vi "AlliGator Get-Set TIFF Series Options.vi"(6 "Set/Get (F)":bool, 8 "error in (no error)":errorcluster, 11 "output cluster in":T1) -> (0 "error out":errorcluster, 3 "output cluster out":T1)   [LabVIEW 2021, in "AlliGator Files.lvlib"]
doc: "Storage of options for dataset export to TIFF series."
uses:
  AlliGator Files.lvlib
  AlliGator TIFF Series Options.ctl
panel:
  # "see the AlliGator License on the block diagram (Ctrl+E or Window:Show Block Diagram)"
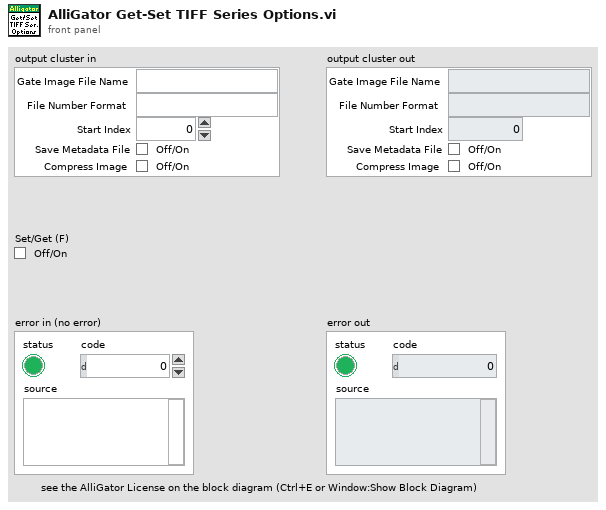
[diagram p1: front panel]
types:
  T1 = typedef "AlliGator Files.lvlib/AlliGator TIFF Series Options.ctl" = cluster{"Gate Image File Name":string, "File Number Format":string, "Start Index":u32, "Save Metadata File":bool, "Compress Image":bool}
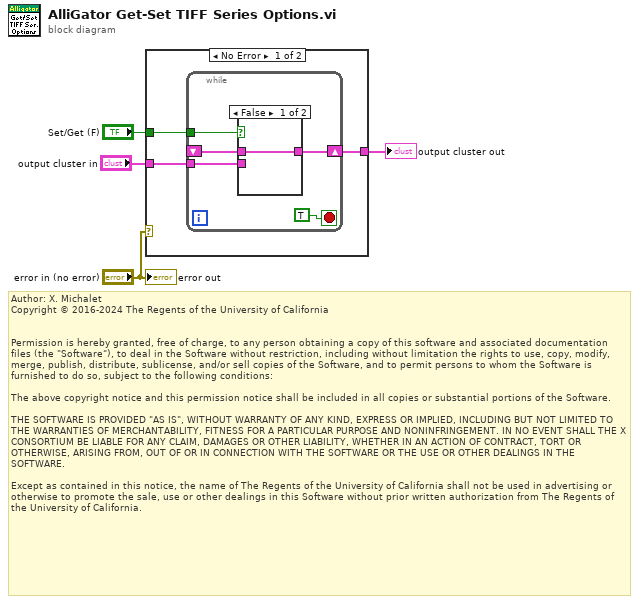
[diagram p0: block diagram]
diagram:
  # "Author: X. Michalet\nCopyright © 2016-2024 The Regents of the University of California\n \n\nPermission is hereby granted, free of charge, to any person obtaining a copy of this software and associated documentation files (the \"Software\"), to deal in the Software without restriction, including without limitation the rights to use, copy, modify, merge, publish, distribute, sublicense, and/or sell copies of the Software, and to permit persons to whom the Software is furnished to do so, subject to the following conditions:\n\nThe above copyright notice and this permission notice shall be included in all copies or substantial portions of the Software.\n\nTHE SOFTWARE IS PROVIDED \"AS IS\", WITHOUT WARRANTY OF ANY KIND, EXPRESS OR IMPLIED, INCLUDING BUT NOT LIMITED TO THE WARRANTIES OF MERCHANTABILITY, FITNESS FOR A PARTICULAR PURPOSE AND NONINFRINGEMENT. IN NO EVENT SHALL THE X CONSORTIUM BE LIABLE FOR ANY CLAIM, DAMAGES OR OTHER LIABILITY, WHETHER IN AN ACTION OF CONTRACT, TORT OR OTHERWISE, ARISING FROM, OUT OF OR IN CONNECTION WITH THE SOFTWARE OR THE USE OR OTHER DEALINGS IN THE SOFTWARE.\n\nExcept as contained in this notice, the name of The Regents of the University of California shall not be used in advertising or otherwise to promote the sale, use or other dealings in this Software without prior written authorization from The Regents of the University of California."
  n1 = case shown="No Error" "error in (no error)" {
    tunnel: "Set/Get (F)" -> [w7 _]
    tunnel: "output cluster in" -> [w6 w15]
    tunnel: [w5 w15] -> w1
    frame No Error {
      n2 = while {
        tunnel: w7 -> [w11]
        shift-right: [w9] -> w5
        shift-left: _ -> [w8]
        tunnel: w6 -> [w10]
        stop <- TRUE stop-if-true
        n3 = case shown="False" w11 {
          tunnel: w10 -> [_ w14]
          tunnel: [w13 w14] -> w9
          tunnel: w8 -> [w13 _]
          frame False {
          }
          frame True {
          }
        }
      }
    }
    frame Error {
    }
  }
  "output cluster out" <- w1
  "error out" <- "error in (no error)"
